vi "Init_odour_bottles.vi"(8 "error in (no error)":errorcluster, 11 "XML Elements":string) -> (0 "error IO":errorcluster, 3 "Array":T1(array[cluster]))   [LabVIEW 2016]
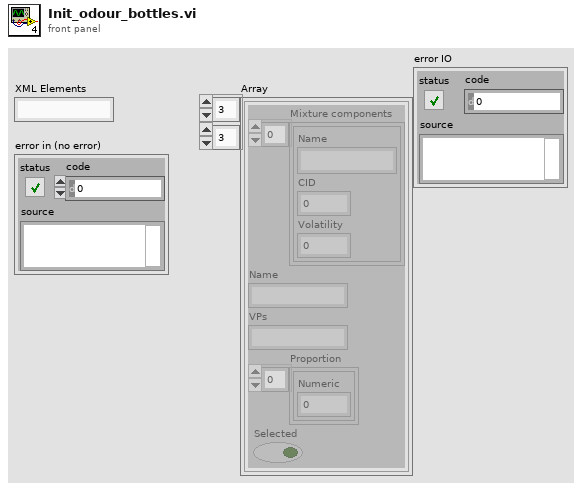
[diagram p1: front panel]
types:
  T1 = cluster{"Mixture components":cluster{"Name":string, "CID":i32, "Volatility":dbl}[], "Name":string, "VPs":string, "Proportion":cluster{"Numeric":dbl}[], "Selected":bool}[][]
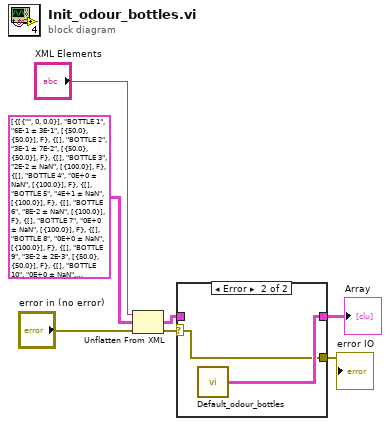
[diagram p0: block diagram]
diagram:
  n1 = Unflatten From XML(xml string="XML Elements", type=T1 [[{"Mixture components"=[{"Name"="", "CID"=0, "Volatility"=0.0}], "Name"="BOTTLE 1", "VPs"="6E-1 ± 3E-1", "Proportion"=[{"Numeric"=50.0}, {"Numeric"=50.0}], "Selected"=FALSE}, {"Mixture components"=[], "Name"="BOTTLE 2", "VPs"="3E-1 ± 7E-2", "Proportion"=[{"Numeric"=50.0}, {"Numeric"=50.0}], "Selected"=FALSE}, {"Mixture components"=[], "Name"="BOTTLE 3", "VPs"="2E-2 ± NaN", "Proportion"=[{"Numeric"=100.0}], "Selected"=FALSE}, {"Mixture components"=[], "Name"="BOTTLE 4", "VPs"="0E+0 ± NaN", "Proportion"=[{"Numeric"=100.0}], "Selected"=FALSE}], [{"Mixture components"=[], "Name"="BOTTLE 5", "VPs"="4E+1 ± NaN", "Proportion"=[{"Numeric"=100.0}], "Selected"=FALSE}, {"Mixture components"=[], "Name"="BOTTLE 6", "VPs"="8E-2 ± NaN", "Proportion"=[{"Numeric"=100.0}], "Selected"=FALSE}, {"Mixture components"=[], "Name"="BOTTLE 7", "VPs"="0E+0 ± NaN", "Proportion"=[{"Numeric"=100.0}], "Selected"=FALSE}, {"Mixture components"=[], "Name"="BOTTLE 8", "VPs"="0E+0 ± NaN", "Proportion"=[{"Numeric"=100.0}], "Selected"=FALSE}], [{"Mixture components"=[], "Name"="BOTTLE 9", "VPs"="3E-2 ± 2E-3", "Proportion"=[{"Numeric"=50.0}, {"Numeric"=50.0}], "Selected"=FALSE}, {"Mixture components"=[], "Name"="BOTTLE 10", "VPs"="0E+0 ± NaN", "Proportion"=[{"Numeric"=100.0}], "Selected"=FALSE}, {"Mixture components"=[], "Name"="BOTTLE 11", "VPs"="5E-2 ± 3E-2", "Proportion"=[{"Numeric"=50.0}, {"Numeric"=50.0}], "Selected"=FALSE}, {"Mixture components"=[], "Name"="BOTTLE 12", "VPs"="4E+0 ± NaN", "Proportion"=[{"Numeric"=100.0}], "Selected"=FALSE}], [{"Mixture components"=[], "Name"="BOTTLE 13", "VPs"="3E+1 ± NaN", "Proportion"=[{"Numeric"=100.0}], "Selected"=FALSE}, {"Mixture components"=[], "Name"="BOTTLE 14", "VPs"="0E+0 ± NaN", "Proportion"=[{"Numeric"=100.0}], "Selected"=FALSE}, {"Mixture components"=[], "Name"="BOTTLE 15", "VPs"="2E-2 ± NaN", "Proportion"=[{"Numeric"=100.0}], "Selected"=FALSE}, {"Mixture components"=[], "Name"="BOTTLE 16", "VPs"="7E-1 ± NaN", "Proportion"=[{"Numeric"=100.0}], "Selected"=FALSE}]] ("Array"), error in (no error)="error in (no error)") -> (value=w7:T1, error out=w6:errorcluster)
  n2 = case shown="Error" w6 {
    selector: w6 -> [w8 w10]
    tunnel: [w9 w11] -> w2
    tunnel: w7 -> [w9 _]
    tunnel: [w8 w10] -> w1
    frame No Error {
    }
    frame Error {
      n3 = call "Default_odour_bottles.vi"() -> ("Array"=w11:T1)
    }
  }
  "Array" <- w2
  "error IO" <- w1
